vi "Agilent 2000 3000 X-Series Harmonics Power Analysis.vi"() -> ()   [LabVIEW 2015]
doc: "This example shows how to apply a Harmonics Power Analysis and read the measurement data."
uses:
  <instrlib>/Agilent 2000 3000 X-Series/Public/Configure/Power Analysis/Configure Power Analysis (Harmonics).vi
  <instrlib>/Agilent 2000 3000 X-Series/Public/Data/Read Measurement (Harmonics Power Analysis).vi
  <instrlib>/Agilent 2000 3000 X-Series/Agilent 2000 3000 X-Series.lvlib
panel:
  out "Power Harmonics Results":string="0"
  out "Ripple Measurement Result":dbl
  in  "Measurement Source 2 (1: Channel 2)":i32(ring)=1 items=["Channel 1", "Channel 2", "Channel 3", "Channel 4", "Math", "Waveform Memory 1", "Waveform Memory 2"]
  in  "Measurement Source 1 (0: Channel 1)":i32(ring) items=["Channel 1", "Channel 2", "Channel 3", "Channel 4", "Math", "Waveform Memory 1", "Waveform Memory 2", "External", "D0", "D1", "D2", "D3", "D4", "D5", "D6", "D7", "D8", "D9", "D10", "D11", "D12", "D13", "D14", "D15"]
  in  "VISA resource name":refnum<visa-resource-name>
  # "(c) 2011-2016 National Instruments.  ALL RIGHTS RESERVED."
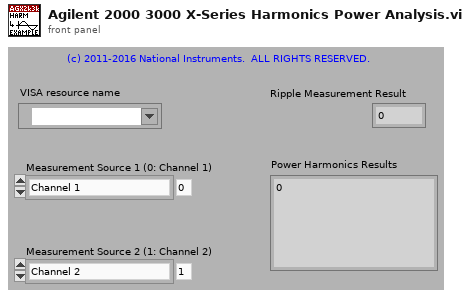
[diagram p1: front panel]
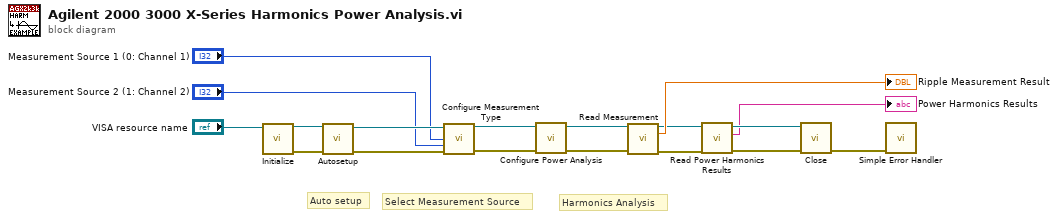
[diagram p0: block diagram]
diagram:
  # "Harmonics Analysis"
  # "Select Measurement Source"
  # "Auto setup"
  n1 = call <instrlib>:"Initialize.vi"("VISA resource name"="VISA resource name") -> ("error out"=w16:errorcluster, "VISA resource name out"=w15:refnum<visa-resource-name>)  [unwired: 4 in, 5 out]
  n2 = call <instrlib>:"Autosetup.vi"("error in (no error)"=w16, "VISA resource name"=w15) -> ("error out"=w13:errorcluster, "VISA resource name out"=w14:refnum<visa-resource-name>)  [unwired: 4 in, 4 out]
  n3 = call <instrlib>:"Configure Measurement Type.vi"("VISA resource name"=w14, "Measurement Source 1 (0: Channel 1)"="Measurement Source 1 (0: Channel 1)", "Measurement Source 2 (1: Channel 2)"="Measurement Source 2 (1: Channel 2)", "error in (no error)"=w13) -> ("VISA resource name out"=w9:refnum<visa-resource-name>, "error out"=w7:errorcluster)  [unwired: 3 in, 7 out]
  n4 = call-poly <instrlib>:"Configure Power Analysis.vi"("error in (no error)"=w7, "VISA resource name"=w9) -> ("error out"=w6:errorcluster, "VISA resource name out"=w8:refnum<visa-resource-name>)  [unwired: 4 in, 4 out]
  n5 = call-poly <instrlib>:"Read Measurement.vi"("VISA resource name"=w8, "error in (no error)"=w6) -> ("VISA resource name out"=w5:refnum<visa-resource-name>, "Harmonics Measurement"=→"Ripple Measurement Result":dbl, "error out"=w4:errorcluster)  [unwired: 1 in, 10 out]
  n6 = call <instrlib>:"Read Power Harmonics Results.vi"("error in (no error)"=w4, "VISA resource name"=w5) -> ("error out"=w2:errorcluster, "Power Harmonics Results"=→"Power Harmonics Results":string, "VISA resource name out"=w3:refnum<visa-resource-name>)  [unwired: 7 out]
  n7 = call <instrlib>:"Close.vi"("error in (no error)"=w2, "VISA resource name"=w3) -> ("error out"=w18:errorcluster)  [unwired: 9 out]
  n8 = call <vilib>:"Simple Error Handler.vi"("error in (no error)"=w18) -> ()  [unwired: 1 in, 8 out]
